vi "Type Cast.vi"() -> ()   [LabVIEW 2020]
panel:
  out "*(type *) &x 3":string
  out "*(type *) &x 2":string
  out "hex integer string":string
  out "number":u32
  out "*(type *) &x":string
  out "Boolean array 2":bool[](array[boolean])
  out "Boolean array":bool[](array[boolean])
  out "Hex 2":u32 format="%8x"
  in  "Numeric 2":sgl=135.9
  out "Numeric":sgl
  in  "Hex":u32=1124591206 format="%8x"
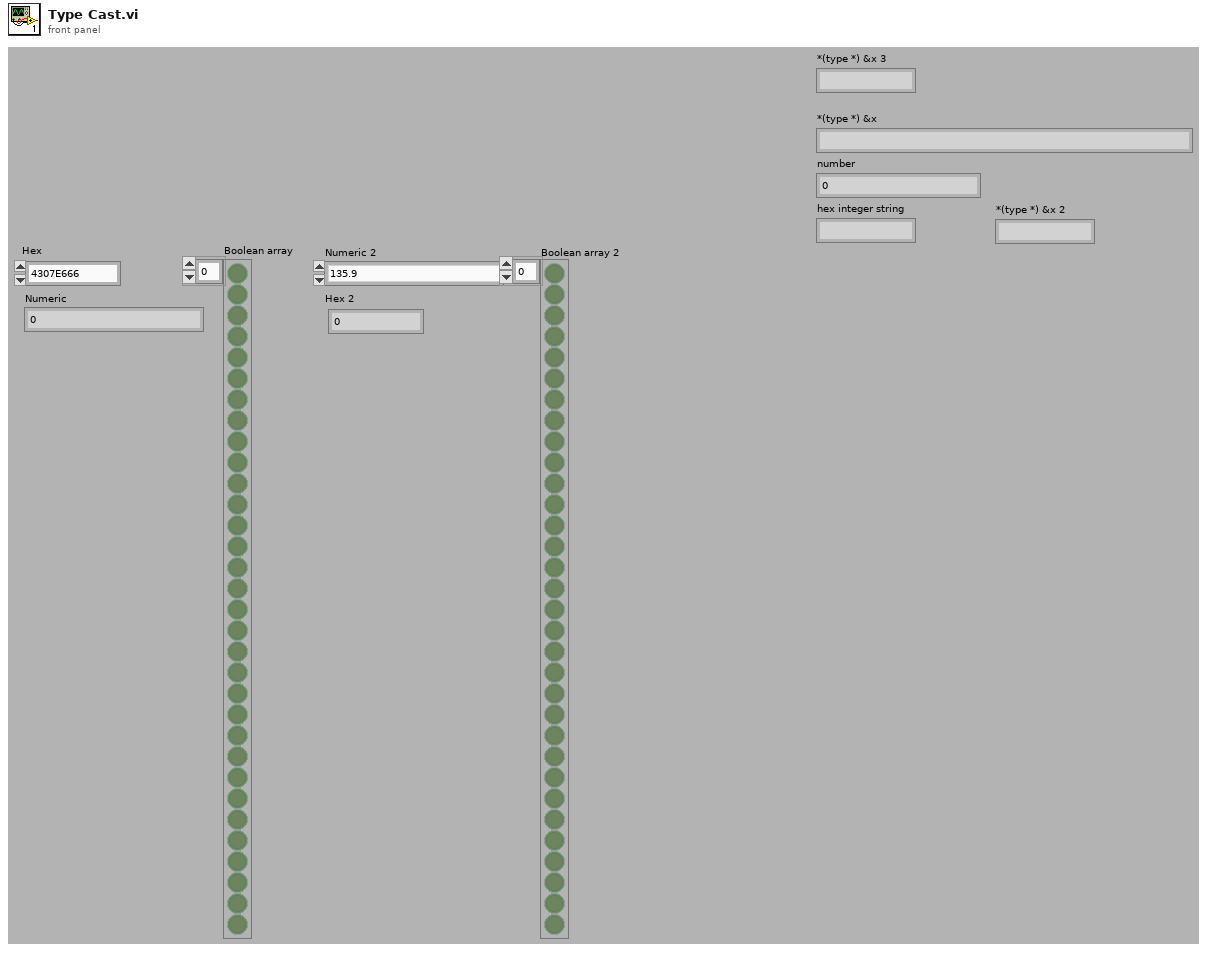
[diagram p1: front panel]
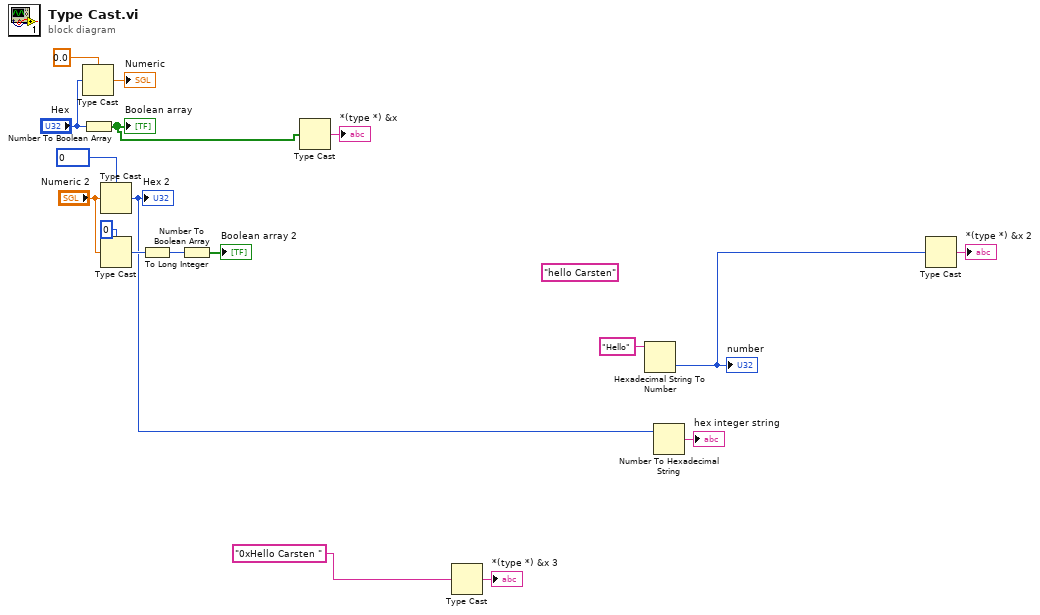
[diagram p0: block diagram]
diagram:
  (unwired) "hello Carsten"
  n1 = Type Cast(type=sgl 0.0 ("Numeric"), x="Hex") -> (*(type *) &x=→"Numeric":sgl)
  n2 = Number To Boolean Array(number="Hex") -> (Boolean array=w9:bool[])
  "Boolean array" <- w9
  n3 = Type Cast(type=u32 0 ("Hex 2"), x="Numeric 2") -> (*(type *) &x=w7:u32)
  "Hex 2" <- w7
  n4 = Type Cast(type=0, x="Numeric 2") -> (*(type *) &x=w12:i32)
  n5 = To Long Integer(number=w12) -> (32bit integer=w13:i32)
  n6 = Number To Boolean Array(number=w13) -> (Boolean array=→"Boolean array 2":bool[])
  n7 = Type Cast(x=w9) -> (*(type *) &x=→"*(type *) &x":string)  [unwired: 1 in]
  n8 = Type Cast(x="0xHello Carsten ") -> (*(type *) &x=→"*(type *) &x 3":string)  [unwired: 1 in]
  n9 = Hexadecimal String To Number(string="Hello") -> (number=w3:u32)  [unwired: 2 in, 1 out]
  "number" <- w3
  n10 = Number To Hexadecimal String(2:w7) -> (0:→"hex integer string":string)  [unwired: 1 in]
  n11 = Type Cast(x=w3) -> (*(type *) &x=→"*(type *) &x 2":string)  [unwired: 1 in]
